vi "setParameters.vi"(10 "Parameters":T1, 11 "StartCommand in":refnum<class "StartCommand.lvclass">) -> (3 "StartCommand out":refnum<class "StartCommand.lvclass">)   [LabVIEW 2016, in "StartCommand.lvclass"]
uses:
  StartCommand.lvclass
  Communicator/Topics/CommandStart.ctl
  Communicator/Topics/CommandId.ctl
  StartCommand.lvclass/StartCommand.ctl
  Communicator/M1M3Communicator.lvlib
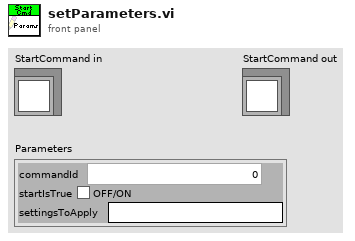
[diagram p1: front panel]
types:
  T1 = typedef "M1M3Communicator.lvlib/CommandStart.ctl" = cluster{"commandId":T2, "startIsTrue":bool, "settingsToApply":string}
  T2 = typedef "M1M3Communicator.lvlib/CommandId.ctl" = i32
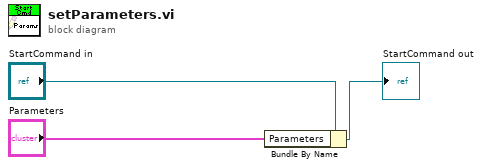
[diagram p0: block diagram]
diagram:
  n1 = Bundle By Name(cluster="StartCommand in", "Parameters"="Parameters") -> (→"StartCommand out":refnum<class "StartCommand.lvclass">)
